vi "DHMS-N.vi"() -> ()   [LabVIEW 2023]
panel:
  out "C":dbl format="%.2f"
  in  "K":dbl format="%#_6f"
  out "%Days":dbl format="%.2f"
  out "%Hours":dbl
  out "Seconds":dbl
  out "Minutes":dbl
  out "Hours":dbl
  out "Days":dbl
  in  "Time s":dbl format="%#_6f"
  in  "?":bool
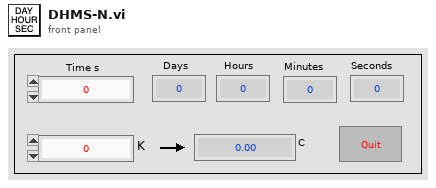
[diagram p1: front panel]
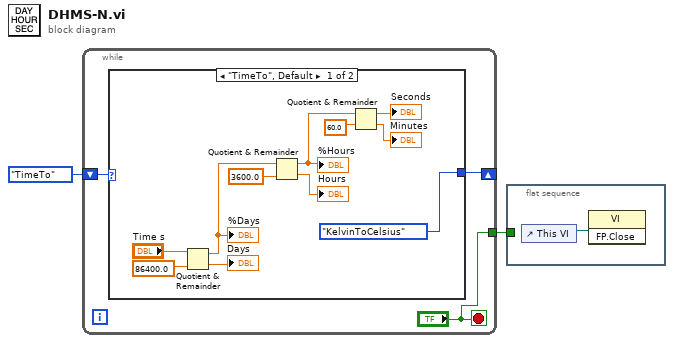
[diagram p0: block diagram]
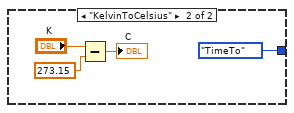
[diagram p2: hidden frame]
diagram:
  n1 = while {
    shift-right: [w3] -> _
    shift-left: enum16{"TimeTo", "KelvinToCelsius"}."TimeTo" -> [w4]
    tunnel: ["?"] -> w2
    stop <- "?" stop-if-true
    n2 = case shown="\"TimeTo\", Default" w4 {
      tunnel: [enum16{"TimeTo", "KelvinToCelsius"}."KelvinToCelsius" enum16{"TimeTo", "KelvinToCelsius"}."TimeTo"] -> w3
      frame "TimeTo", Default {
        n3 = Quotient & Remainder(x="Time s", y=86400.0) -> (x-y*floor(x/y)=w13:dbl, floor(x/y)=→"Days":dbl)
        "%Days" <- w13
        n4 = Quotient & Remainder(x=w13, y=3600.0) -> (x-y*floor(x/y)=w10:dbl, floor(x/y)=→"Hours":dbl)
        "%Hours" <- w10
        n5 = Quotient & Remainder(x=w10, y=60.0) -> (x-y*floor(x/y)=→"Seconds":dbl, floor(x/y)=→"Minutes":dbl)
      }
      frame "KelvinToCelsius" {
        n6 = Subtract(x="K", y=273.15) -> (x-y=→"C":dbl)
      }
    }
  }
  n7 = flat-sequence {
    tunnel: w2 -> [_]
    frame #0 {
      n8 = control-ref of="This VI"() -> (w21:refnum<vi>)
      n9 = invoke class="VI" method="FP.Close"(reference=w21) -> ()  [unwired: 2 in, 3 out]
    }
  }
